vi "days since 1900.vi"() -> (3 "fractional days":ext)   [LabVIEW 2012]
panel:
  out "current time":timestamp
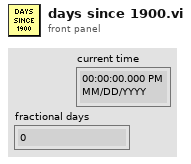
[diagram p1: front panel]
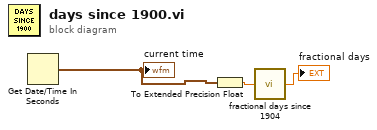
[diagram p0: block diagram]
diagram:
  n1 = Get Date/Time In Seconds() -> (seconds since 1Jan1904=w3:timestamp)
  "current time" <- w3
  n2 = To Extended Precision Float(1:w3) -> (0:w2:ext)
  n3 = call "fractional days since 1904.vi"("seconds since 1904"=w2) -> ("Days"=→"fractional days":dbl)
